vi "TDTSyn-Get Events.vi"(0 "State In":T1, 9 "Max Read":i32=20000, 11 "error in (no error)":errorcluster) -> (4 "State Out":T1, 8 "Events":dbl[][](array[numeric]), 10 "backlog":bool, 15 "error out":errorcluster)   [LabVIEW 2020]
uses:
  TDTSyn-State.ctl
  PXI DAQ VIs/Utility VIs/Array Dimensions (2D).vi
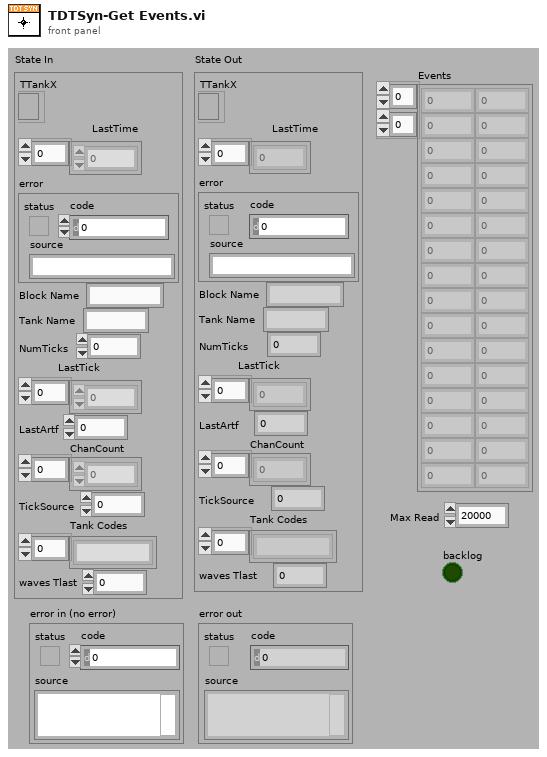
[diagram p1: front panel]
types:
  T1 = typedef "TDTSyn-State.ctl" = cluster{"TTankX":refnum<k7>, "LastTime":dbl[], "error":errorcluster, "Block Name":string, "Tank Name":string, "NumTicks":i32, "LastTick":dbl[], "LastArtf":dbl, "ChanCount":i32[], "TickSource":i32, "Tank Codes":string[], "waves Tlast":dbl}
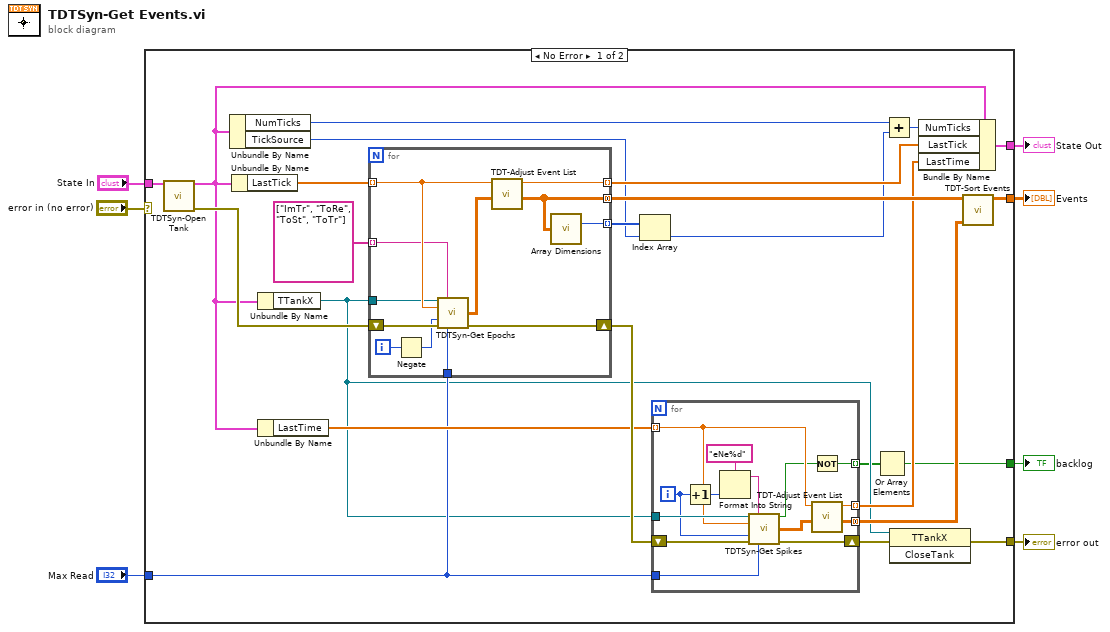
[diagram p0: block diagram]
diagram:
  n1 = case shown="No Error" "error in (no error)" {
    selector: "error in (no error)" -> [_ w59]
    tunnel: [w19 w59] -> w6
    tunnel: "State In" -> [w24 w58]
    tunnel: "Max Read" -> [w21 _]
    tunnel: [w26 _] -> w3
    tunnel: [w29 w58] -> w2
    tunnel: [w9 _] -> w1
    frame No Error {
      n2 = call "TDTSyn-Open Tank.vi"("State In"=w24) -> ("State Out"=w12:T1, "error out"=w25:errorcluster)  [unwired: 13 in]
      n3 = Unbundle By Name(w12) -> ("NumTicks"=w30:i32, "TickSource"=w15:i32)
      n4 = Unbundle By Name(w12) -> ("LastTick"=w23:dbl[])
      n5 = Unbundle By Name(w12) -> ("TTankX"=w11:refnum<k7>)
      n6 = Unbundle By Name(w12) -> ("LastTime"=w22:dbl[])
      n7 = for {
        tunnel: [w42] -> w27 mode=indexing
        tunnel: w23 -> [w39] mode=indexing
        tunnel: w21 -> [w38]
        tunnel: w11 -> [w37]
        tunnel: [w33] -> w18 mode=concatenating
        shift-right: [w43] -> w31
        shift-left: w25 -> [w40]
        tunnel: string[] ["ImTr", "ToRe", "ToSt", "ToTr"] ("Epoch code") -> [w36] mode=indexing
        tunnel: [w32] -> w17 mode=indexing
        i -> [w35]
        n8 = Negate(x=w35) -> (-x=w34:i32)
        n9 = call "TDTSyn-Get Epochs.vi"("TTankX"=w37, "Epoch code"=w36, "T1"=w39, "code"=w34, "error in (no error)"=w40, "Max Read"=w38) -> ("Epoch times"=w41:dbl[][], "error out"=w43:errorcluster)  [unwired: 6 in, 2 out]
        n10 = call "TDT-Adjust Event List.vi"("Events in"=w41, "Last In"=w39) -> ("Events out"=w33:dbl[][], "Last out"=w42:dbl)  [unwired: 8 in]
        n11 = call-poly "Array Dimensions.vi"("2D Array"=w33) -> ("# rows"=w32:i32)  [unwired: 13 in, 1 out]
      }
      n12 = Index Array(array=w17, index=w15) -> (element=w16:i32)
      n13 = for {
        tunnel: w22 -> [w48] mode=indexing
        tunnel: w21 -> [w56]
        tunnel: w11 -> [w54]
        shift-right: [w55] -> w20
        shift-left: w31 -> [w57]
        tunnel: [w47] -> w14 mode=indexing
        tunnel: [w46] -> w13 mode=concatenating
        tunnel: [w44] -> w10 mode=indexing
        i -> [w52]
        n14 = Increment(x=w52) -> (x+1=w50:i32)
        n15 = Format Into String(format string="eNe%d", w50) -> (resulting string=w53:string)  [unwired: 2 in, 1 out]
        n16 = call "TDTSyn-Get Spikes.vi"("TTankX"=w54, "TankCode"=w53, "T1"=w48, "offset"=w52, "error in (no error)"=w57, "Max Read"=w56) -> ("Got 'em all"=w45:bool, "Spike times"=w49:dbl[][], "error out"=w55:errorcluster)  [unwired: 6 in, 1 out]
        n17 = Not(x=w45) -> (.not. x?=w44:bool)
        n18 = call "TDT-Adjust Event List.vi"("Events in"=w49, "Last In"=w48) -> ("Events out"=w46:dbl[][], "Last out"=w47:dbl)  [unwired: 8 in]
      }
      n19 = Or Array Elements(Boolean array=w10) -> (logical OR=w9:bool)
      n20 = Add(x=w30, y=w16) -> (x+y=w28:i32)
      n21 = invoke class="TTankX" method="CloseTank"(reference=w11, error in=w20) -> (error out=w19:errorcluster)  [unwired: 1 in, 2 out]
      n22 = Bundle By Name(cluster=w12, "NumTicks"=w28, "LastTick"=w27, "LastTime"=w14) -> (w29:T1)
      n23 = call "TDT-Sort Events.vi"("Tosca Markers"=w13, "Ticks"=w18) -> ("Sorted events"=w26:dbl[][])  [unwired: 9 in]
    }
    frame Error {
    }
  }
  "error out" <- w6
  "State Out" <- w2
  "Events" <- w3
  "backlog" <- w1
